vi "cicrulo.vi"() -> ()   [LabVIEW 2020]
panel:
  out "Gráfico de un círculo":cluster{dbl[], dbl[]}(graph)
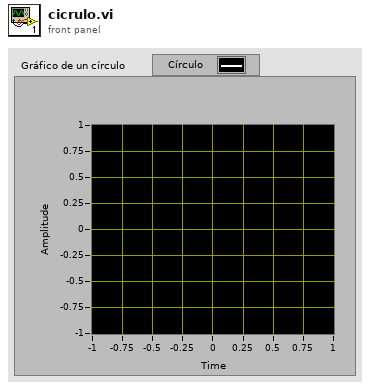
[diagram p1: front panel]
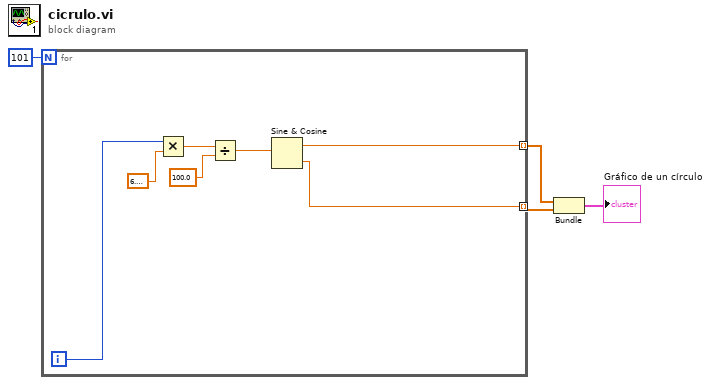
[diagram p0: block diagram]
diagram:
  n1 = for {
    N: 101 -> [_]
    tunnel: [w6] -> w2 mode=indexing
    tunnel: [w5] -> w3 mode=indexing
    i -> [w8]
    n2 = Multiply(x=w8, y=6.283185307179586) -> (x*y=w10:dbl)
    n3 = Divide(x=w10, y=100.0) -> (x/y=w7:dbl)
    n4 = Sine & Cosine(0:w7) -> (1:w5:dbl, 2:w6:dbl)
  }
  n5 = Bundle(w3, w2) -> (→"Gráfico de un círculo":cluster{dbl[], dbl[]})  [unwired: 1 in]
